vi "Fixed Number Table Read.vi"(8 "error in":errorcluster, 9 "Data to read in":T2, 10 "Channel_Timing in":T1, 11 "Report Viewer in":refnum<class "Report Viewer.lvclass">) -> (0 "error out":errorcluster, 1 "Data to read out":T2, 2 "Channel_Timing out":T1, 3 "Report Viewer out":refnum<class "Report Viewer.lvclass">, 4 "Table Data":string[](array[string]), 6 "Table_Header":string[](array[string]))   [LabVIEW 2019, in "Report Viewer.lvlib" / "Report Viewer.lvclass"]
uses:
  Library/Report Viewer.lvclass
  Custom Controls/Data to Read.ctl
  Custom Controls/Channel_Timing.ctl
  Library/Report Viewer.lvclass/Report Viewer.ctl
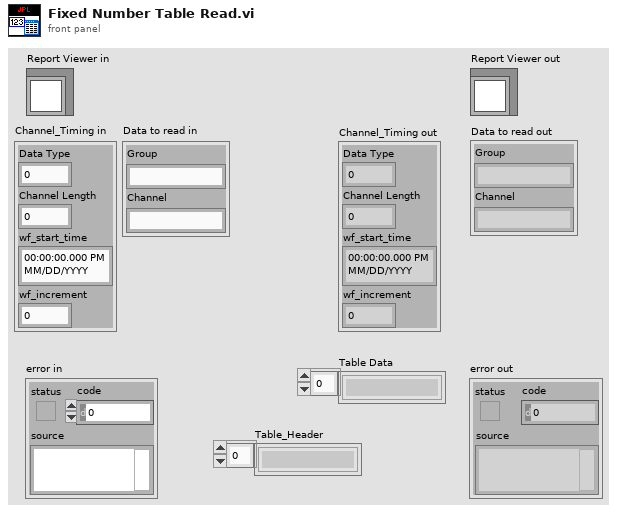
[diagram p1: front panel]
types:
  T1 = typedef "Report Viewer.lvlib/Report Viewer.lvclass/Channel_Timing.ctl" = cluster{"Data Type":u16, "Channel Length":u64, "wf_start_time":timestamp, "wf_increment":dbl}
  T2 = typedef "Report Viewer.lvlib/Report Viewer.lvclass/Data to Read.ctl" = cluster{"Group":string, "Channel":string}
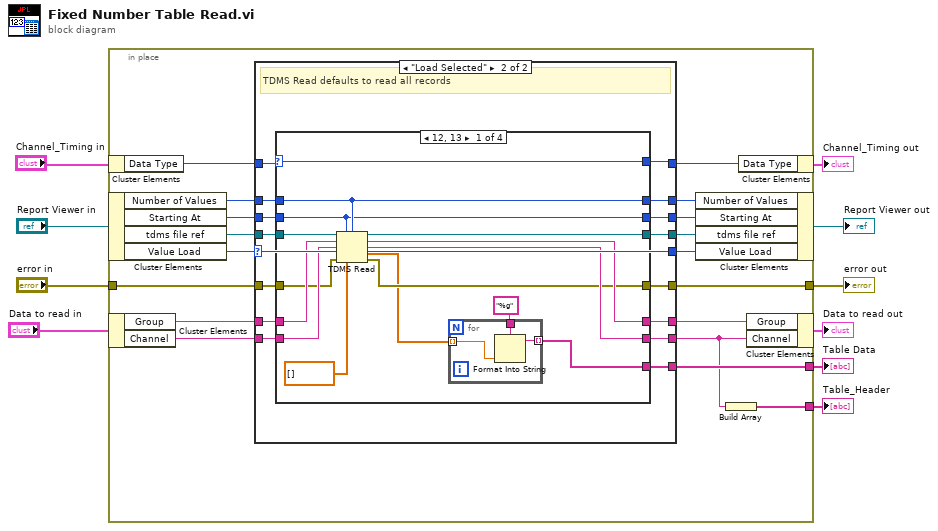
[diagram p0: block diagram]
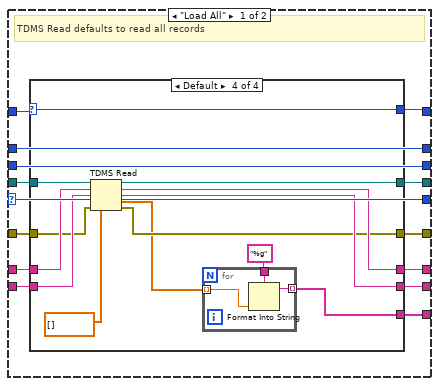
[diagram p2: hidden frame]
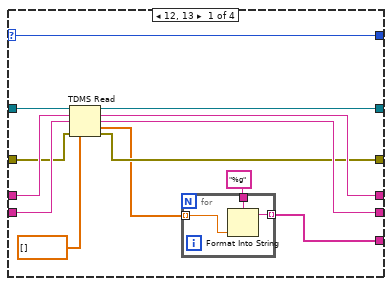
[diagram p3: hidden frame]
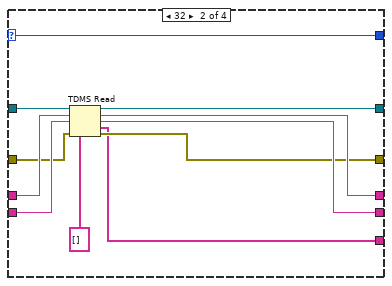
[diagram p4: hidden frame]
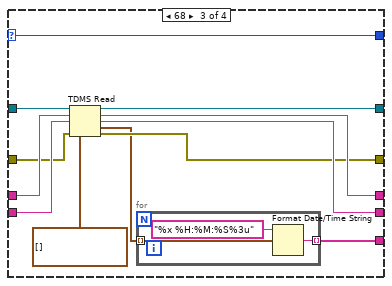
[diagram p5: hidden frame]
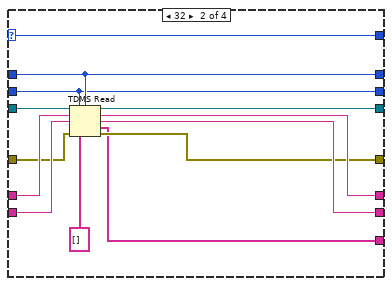
[diagram p6: hidden frame]
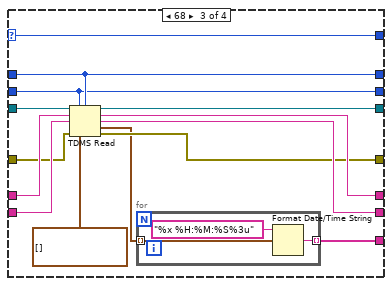
[diagram p7: hidden frame]
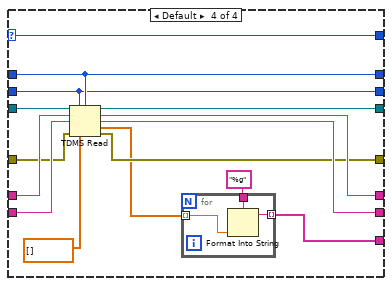
[diagram p8: hidden frame]
diagram:
  n1 = in-place {
    in-place-border: "error in" -> [w16]
    in-place-border: [w14] -> w5
    in-place-border: [w13] -> w4
    in-place-border: [w11] -> w1
    n2 = in-place-cluster #1("Channel_Timing in") -> ("Data Type"=w24:u16)
    n3 = in-place-cluster #2("Report Viewer in") -> ("Number of Values"=w26:i32, "Starting At"=w25:i32, "tdms file ref"=w27:refnum<k34>, "Value Load"=w28:enum32{"Load All", "Load Selected"})
    n4 = in-place-cluster #3("Data to read in") -> ("Group"=w19:string, "Channel"=w18:string)
    n5 = case shown="\"Load Selected\"" w28 {
      selector: w28 -> [w36 w112]
      tunnel: w27 -> [w41 w115]
      tunnel: w26 -> [w40 w103]
      tunnel: w25 -> [w39 w104]
      tunnel: w24 -> [w42 w116]
      tunnel: [w38 w114] -> w23
      tunnel: [w40 w102] -> w22
      tunnel: [w39 w101] -> w21
      tunnel: [w36 w112] -> w20
      tunnel: w19 -> [w35 w111]
      tunnel: w18 -> [w34 w110]
      tunnel: [w33 w109] -> w17
      tunnel: [w32 w108] -> w12
      tunnel: w16 -> [w31 w107]
      tunnel: [w37 w113] -> w15
      tunnel: [w30 w106] -> w14
      tunnel: [w29 w105] -> w13
      frame "Load All" {
        # "TDMS Read defaults to read all records"
        n6 = case shown="Default" w42 {
          selector: w42 -> [w54 w68 w80 w96]
          tunnel: w41 -> [w55 w69 w81 w97]
          tunnel: [w54 w68 w80 w96] -> w38
          tunnel: [w53 w67 w79 w95] -> w37
          tunnel: w35 -> [w52 w66 w78 w94]
          tunnel: w34 -> [w51 w65 w77 w93]
          tunnel: [w50 w64 w76 w92] -> w33
          tunnel: [w49 w63 w75 w91] -> w32
          tunnel: w31 -> [w48 w62 w74 w90]
          tunnel: [w47 w61 w73 w89] -> w30
          tunnel: [w44 w59 w70 w85] -> w29
          frame 12, 13 {
            n7 = TDMS Read(0:w55, 5:w52, 7:w51, 11:w48, 12:cdb[] []) -> (4:w53:refnum<k34>, 6:w50:string, 8:w49:string, 10:w45:cdb[], 15:w47:errorcluster)  [unwired: 3 in, 1 out]
            n8 = for {
              tunnel: "%g" ("format string") -> [w58]
              tunnel: w45 -> [w57] mode=indexing
              tunnel: [w56] -> w44 mode=indexing
              n9 = Format Into String(format string=w58, w57) -> (resulting string=w56:string)  [unwired: 2 in, 1 out]
            }
          }
          frame 32 {
            n10 = TDMS Read(0:w69, 5:w66, 7:w65, 11:w62, 12:string[] []) -> (4:w67:refnum<k34>, 6:w64:string, 8:w63:string, 10:w59:string[], 15:w61:errorcluster)  [unwired: 3 in, 1 out]
          }
          frame 68 {
            n11 = TDMS Read(0:w81, 5:w78, 7:w77, 11:w74, 12:timestamp[] []) -> (4:w79:refnum<k34>, 6:w76:string, 8:w75:string, 10:w71:timestamp[], 15:w73:errorcluster)  [unwired: 3 in, 1 out]
            n12 = for {
              tunnel: [w84] -> w70 mode=indexing
              tunnel: w71 -> [w83] mode=indexing
              n13 = Format Date/Time String(time format string (%c)="%x %H:%M:%S%3u", seconds (now)=w83) -> (date/time string=w84:string)  [unwired: 1 in]
            }
          }
          frame Default {
            n14 = TDMS Read(0:w97, 5:w94, 7:w93, 11:w90, 12:dbl[] []) -> (4:w95:refnum<k34>, 6:w92:string, 8:w91:string, 10:w86:dbl[], 15:w89:errorcluster)  [unwired: 3 in, 1 out]
            n15 = for {
              tunnel: "%g" ("format string") -> [w100]
              tunnel: w86 -> [w99] mode=indexing
              tunnel: [w98] -> w85 mode=indexing
              n16 = Format Into String(format string=w100, w99) -> (resulting string=w98:string)  [unwired: 2 in, 1 out]
            }
          }
        }
      }
      frame "Load Selected" {
        # "TDMS Read defaults to read all records"
        n17 = case shown="12, 13" w116 {
          selector: w116 -> [w130 w146 w160 w178]
          tunnel: w115 -> [w131 w147 w161 w179]
          tunnel: [w130 w146 w160 w178] -> w114
          tunnel: [w129 w145 w159 w177] -> w113
          tunnel: w111 -> [w128 w144 w158 w176]
          tunnel: w110 -> [w127 w143 w157 w175]
          tunnel: [w126 w142 w156 w174] -> w109
          tunnel: [w125 w141 w155 w173] -> w108
          tunnel: w107 -> [w124 w140 w154 w172]
          tunnel: [w123 w139 w153 w171] -> w106
          tunnel: [w120 w137 w150 w167] -> w105
          tunnel: w104 -> [w117 w135 w148 w165]
          tunnel: w103 -> [w118 w136 w149 w166]
          tunnel: [w118 w136 w149 w166] -> w102
          tunnel: [w117 w135 w148 w165] -> w101
          frame 12, 13 {
            n18 = TDMS Read(0:w131, 1:w117, 2:w118, 5:w128, 7:w127, 11:w124, 12:cdb[] []) -> (4:w129:refnum<k34>, 6:w126:string, 8:w125:string, 10:w121:cdb[], 15:w123:errorcluster)  [unwired: 1 in, 1 out]
            n19 = for {
              tunnel: "%g" ("format string") -> [w134]
              tunnel: w121 -> [w133] mode=indexing
              tunnel: [w132] -> w120 mode=indexing
              n20 = Format Into String(format string=w134, w133) -> (resulting string=w132:string)  [unwired: 2 in, 1 out]
            }
          }
          frame 32 {
            n21 = TDMS Read(0:w147, 1:w135, 2:w136, 5:w144, 7:w143, 11:w140, 12:string[] []) -> (4:w145:refnum<k34>, 6:w142:string, 8:w141:string, 10:w137:string[], 15:w139:errorcluster)  [unwired: 1 in, 1 out]
          }
          frame 68 {
            n22 = TDMS Read(0:w161, 1:w148, 2:w149, 5:w158, 7:w157, 11:w154, 12:timestamp[] []) -> (4:w159:refnum<k34>, 6:w156:string, 8:w155:string, 10:w151:timestamp[], 15:w153:errorcluster)  [unwired: 1 in, 1 out]
            n23 = for {
              tunnel: [w164] -> w150 mode=indexing
              tunnel: w151 -> [w163] mode=indexing
              n24 = Format Date/Time String(time format string (%c)="%x %H:%M:%S%3u", seconds (now)=w163) -> (date/time string=w164:string)  [unwired: 1 in]
            }
          }
          frame Default {
            n25 = TDMS Read(0:w179, 1:w165, 2:w166, 5:w176, 7:w175, 11:w172, 12:dbl[] []) -> (4:w177:refnum<k34>, 6:w174:string, 8:w173:string, 10:w168:dbl[], 15:w171:errorcluster)  [unwired: 1 in, 1 out]
            n26 = for {
              tunnel: "%g" ("format string") -> [w182]
              tunnel: w168 -> [w181] mode=indexing
              tunnel: [w180] -> w167 mode=indexing
              n27 = Format Into String(format string=w182, w181) -> (resulting string=w180:string)  [unwired: 2 in, 1 out]
            }
          }
        }
      }
    }
    n28 = in-place-cluster #2("Number of Values"=w22, "Starting At"=w21, "tdms file ref"=w15, "Value Load"=w20) -> (→"Report Viewer out":refnum<class "Report Viewer.lvclass">)
    n29 = Build Array(w12) -> (w11:string[])
    n30 = in-place-cluster #1("Data Type"=w23) -> (→"Channel_Timing out":T1)
    n31 = in-place-cluster #3("Group"=w17, "Channel"=w12) -> (→"Data to read out":T2)
  }
  "error out" <- w5
  "Table Data" <- w4
  "Table_Header" <- w1
